vi "Code2Ps.vi"(10 "Code2 In":string, 11 "Data In":T1) -> (3 "Data Out":T1)   [LabVIEW 2014]
uses:
  controls/Data1.ctl
panel:
  # "ら      戳"
  # "诀       贺"
  # "诀       腹"
  # "°Ó«~±ø½X"
  # "OK"
  # "¥x"
  # "NG"
  # "¥x"
  # "Á`­p"
  # "¥x"
  # "ら      戳"
  # "诀       贺"
  # "诀       腹"
  # "°Ó«~±ø½X"
  # "OK"
  # "¥x"
  # "NG"
  # "¥x"
  # "Á`­p"
  # "¥x"
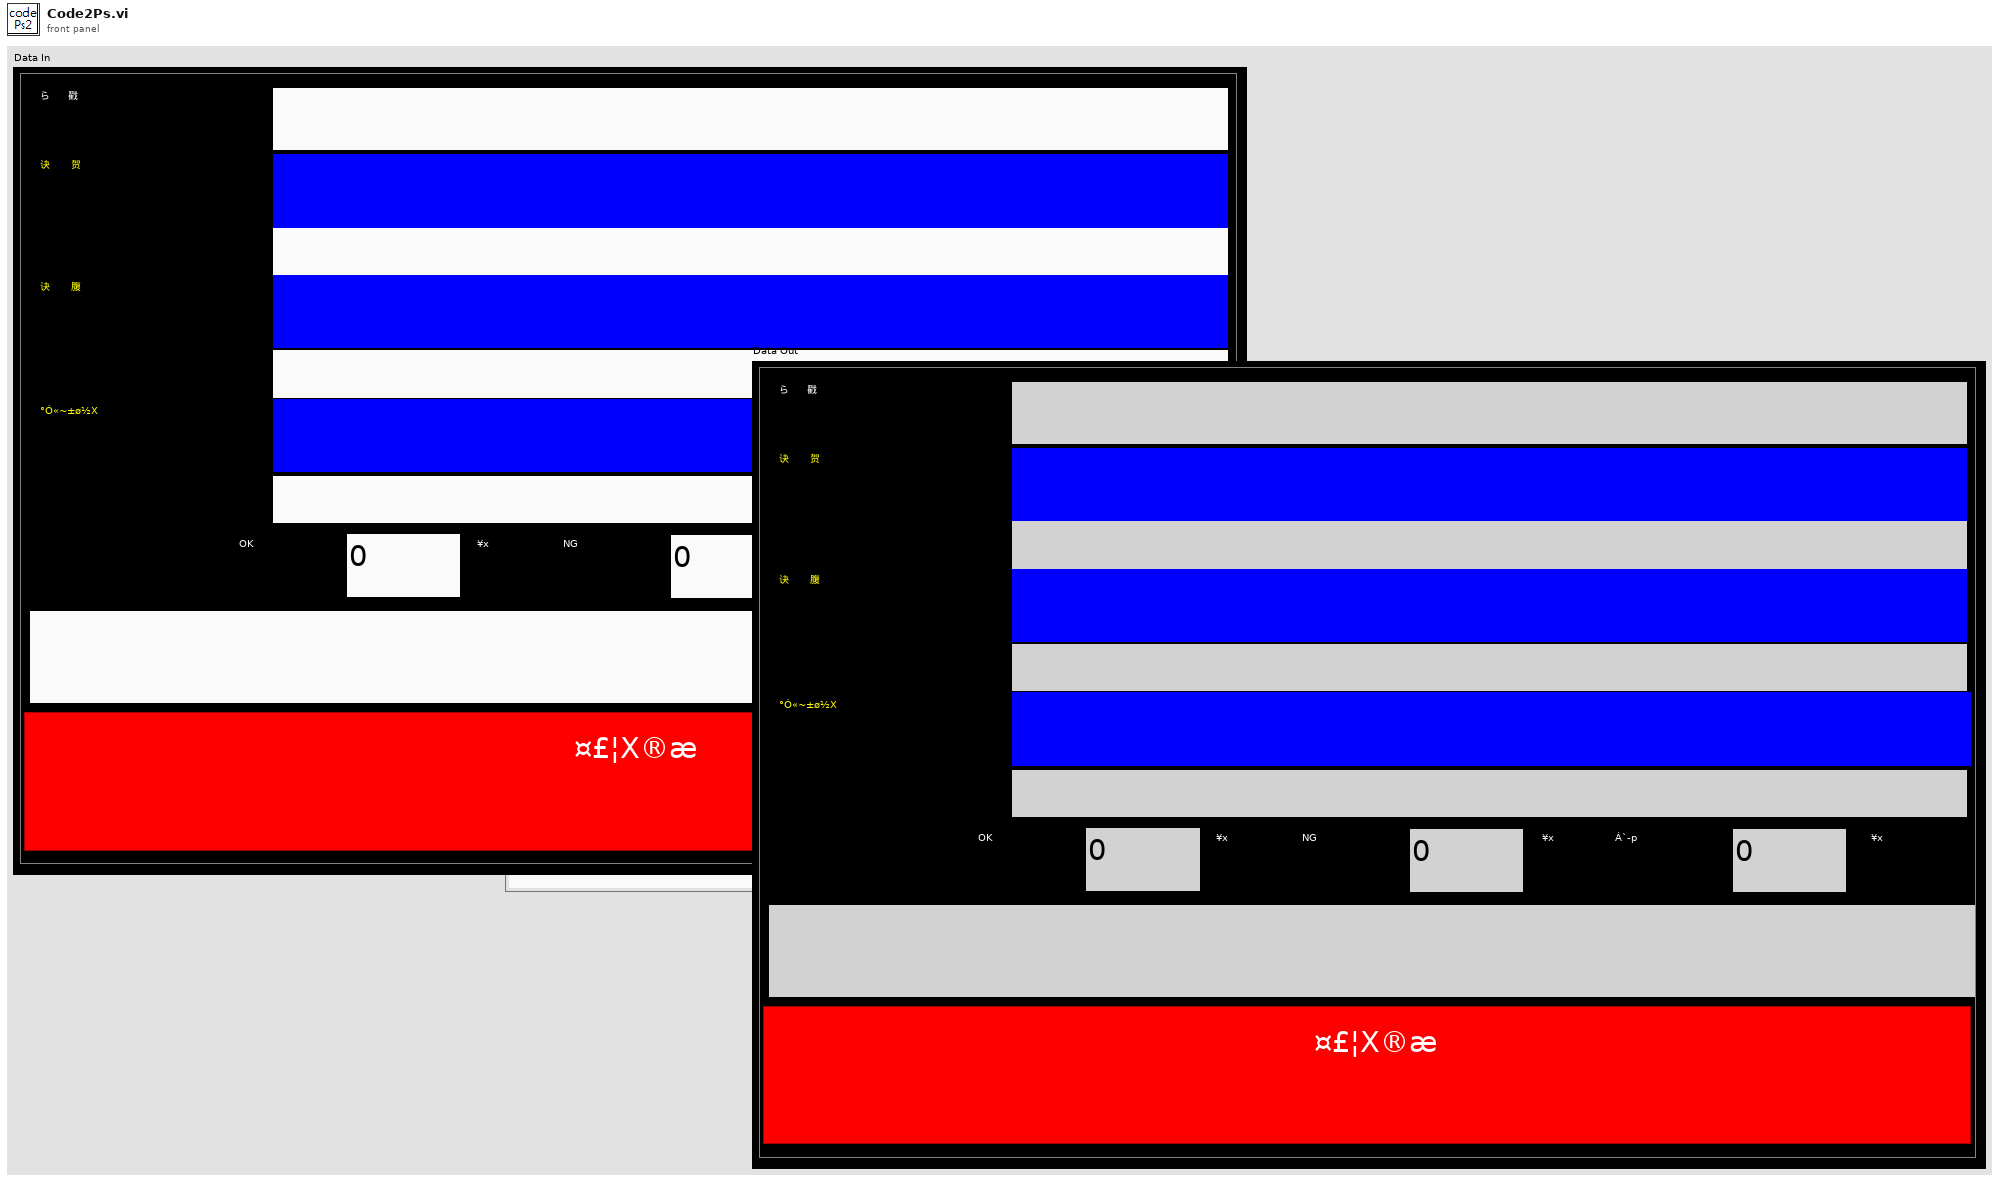
[diagram p1: front panel]
types:
  T1 = typedef "Data1.ctl" = cluster{"Date":string, "BarCode1":string, "BarCode2":string, "BarCode3":string, "Message":string, "OK Count":u16, "NG Count":u16, "Total Count":u16, "ModelData":string[][], "OK&NG":bool, "COM1":refnum<visa-resource-name>, "COM2":refnum<visa-resource-name>, "IO":i32, "Time":u32, "TCP":refnum<k5>, "TCP 2":refnum<k5>, "COM1 2":refnum<visa-resource-name>, "CheckPars":string, "BarCode1_1":string, "BarCode2_1":string, "BarCode3_1":string}
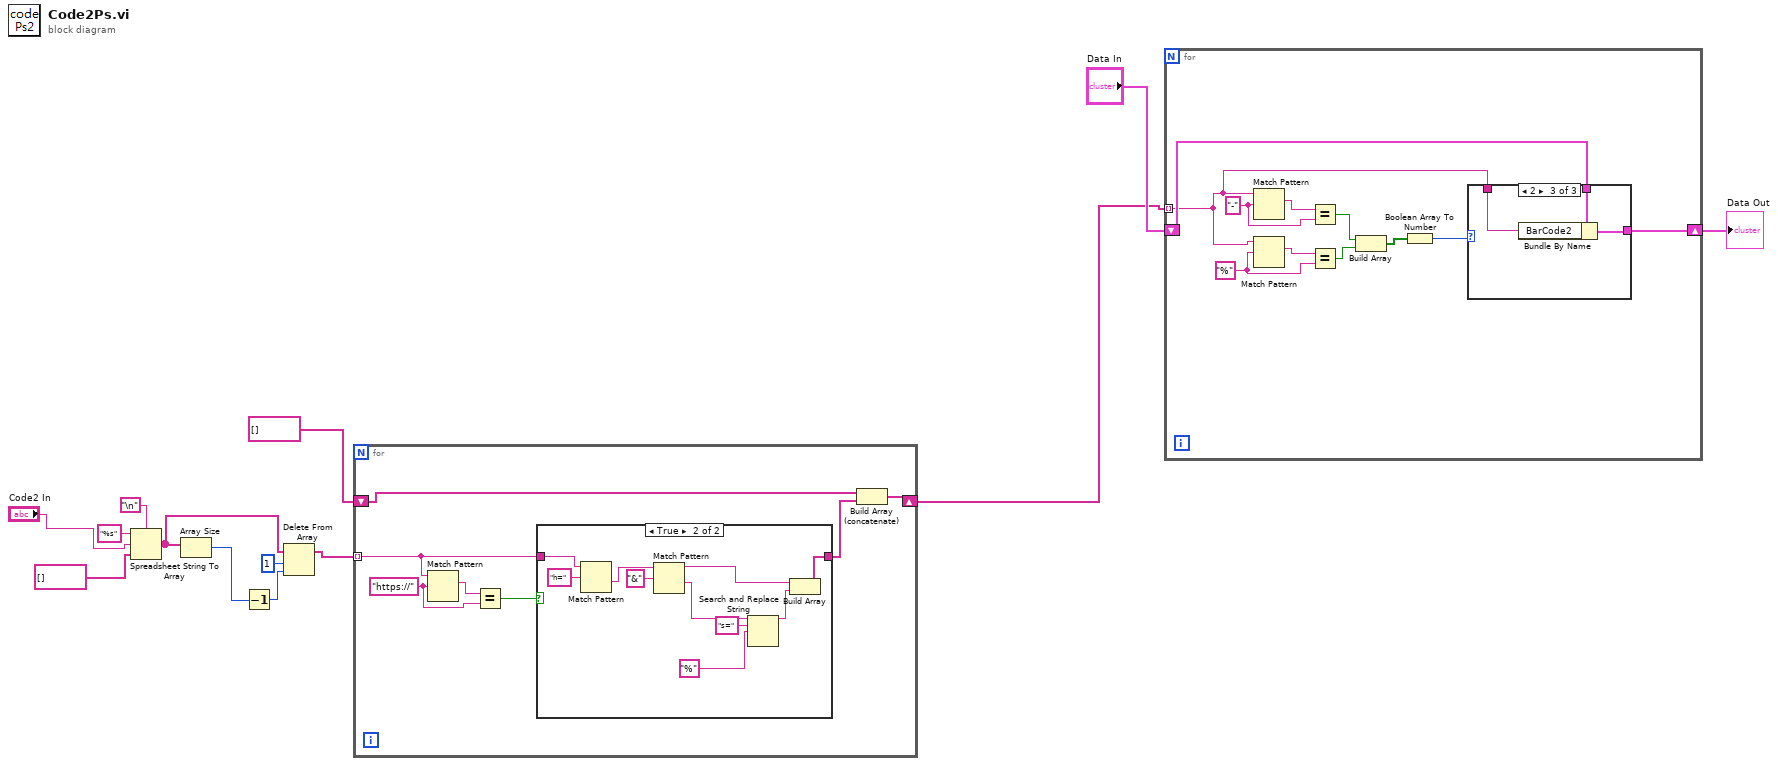
[diagram p0: block diagram]
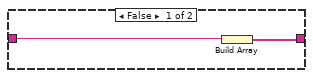
[diagram p2: hidden frame]
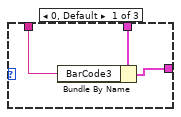
[diagram p3: hidden frame]
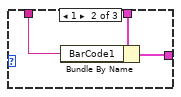
[diagram p4: hidden frame]
diagram:
  n1 = Spreadsheet String To Array(delimiter (Tab)="\n", format string="%s", spreadsheet string="Code2 In", array type (2D Dbl)=string[] []) -> (array=w8:string[])
  n2 = Array Size(array=w8) -> (size(s)=w6:i32)
  n3 = Decrement(x=w6) -> (x-1=w5:i32)
  n4 = Delete From Array(array=w8, length=1, index=w5) -> (array with subset deleted=w2:string[])  [unwired: 1 out]
  n5 = for {
    tunnel: w2 -> [w17] mode=indexing
    shift-right: [w16] -> w1
    shift-left: string[] [] -> [w14]
    w19 = "https://" ("regular expression")
    n6 = Match Pattern(string=w17, regular expression=w19) -> (match substring=w18:string)  [unwired: 1 in, 3 out]
    n7 = Equal?(x=w18, y=w19) -> (x = y?=w20:bool)
    n8 = case shown="True" w20 {
      tunnel: [w21 w24] -> w15
      tunnel: w17 -> [w22 w23]
      frame False {
        n9 = Build Array(w22) -> (w21:string[])
      }
      frame True {
        n10 = Match Pattern(string=w23, regular expression="h=") -> (after substring=w26:string)  [unwired: 1 in, 3 out]
        n11 = Match Pattern(string=w26, regular expression="&") -> (before substring=w28:string, after substring=w29:string)  [unwired: 1 in, 2 out]
        n12 = Search and Replace String(input string=w29, search string="s=", replace string="%" ("replace string (\"\")")) -> (result string=w32:string)  [unwired: 5 in, 3 out]
        n13 = Build Array(w28, w32) -> (w24:string[])
      }
    }
    n14 = Build Array (concatenate)(w14, w15) -> (w16:string[])
  }
  n15 = for {
    shift-right: [w34] -> w12
    shift-left: "Data In" -> [w35]
    tunnel: w1 -> [w33] mode=indexing
    w40 = "%" ("regular expression")
    w42 = "-" ("regular expression")
    n16 = Match Pattern(string=w33, regular expression=w42) -> (match substring=w43:string)  [unwired: 1 in, 3 out]
    n17 = Match Pattern(string=w33, regular expression=w40) -> (match substring=w41:string)  [unwired: 1 in, 3 out]
    n18 = Equal?(x=w43, y=w42) -> (x = y?=w39:bool)
    n19 = Equal?(x=w41, y=w40) -> (x = y?=w38:bool)
    n20 = Build Array(w39, w38) -> (w37:bool[])
    n21 = Boolean Array To Number(Boolean array=w37) -> (number=w36:u32)
    n22 = case shown="2" w36 {
      tunnel: w33 -> [w46 w47 w50]
      tunnel: w35 -> [w45 w49 w52]
      tunnel: [w44 w48 w51] -> w34
      frame 0, Default {
        n23 = Bundle By Name(cluster=w45, "BarCode3"=w46) -> (w44:T1)
      }
      frame 1 {
        n24 = Bundle By Name(cluster=w49, "BarCode1"=w47) -> (w48:T1)
      }
      frame 2 {
        n25 = Bundle By Name(cluster=w52, "BarCode2"=w50) -> (w51:T1)
      }
    }
  }
  "Data Out" <- w12
